vi "checksum.vi"(8 "error in (no error)":errorcluster, 10 "input":string, 11 "Tektronix RSA5106A in":refnum<class "Tektronix RSA5106A.lvclass">) -> (0 "error out":errorcluster, 2 "output":string, 3 "Tektronix RSA5106A out":refnum<class "Tektronix RSA5106A.lvclass">)   [LabVIEW 2013, in "Tektronix RSA5106A.lvclass"]
uses:
  Tektronix RSA5106A.lvclass
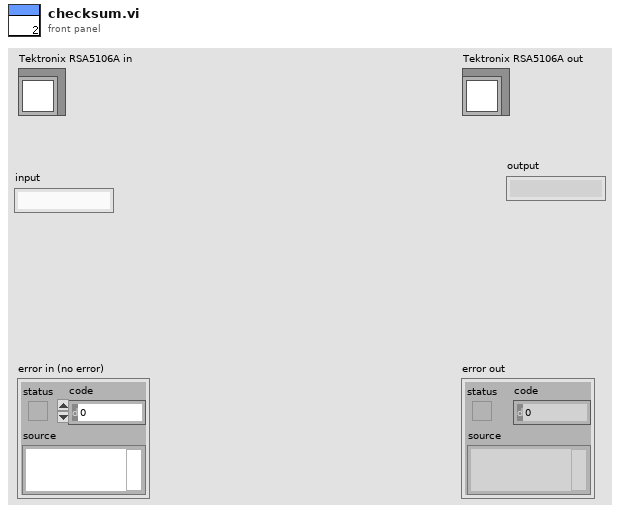
[diagram p1: front panel]
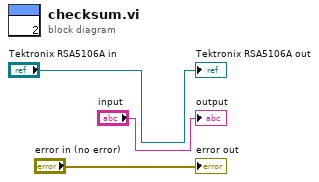
[diagram p0: block diagram]
diagram:
  "error out" <- "error in (no error)"
  "Tektronix RSA5106A out" <- "Tektronix RSA5106A in"
  "output" <- "input"
